vi "Shift_008.vi"() -> ()   [LabVIEW 2019]
uses:
  <vilib>/Utility/file.llb/Write Delimited Spreadsheet (DBL).vi
panel:
  out "path":path
  out "Force Chart":cluster{dbl[unit], dbl[unit]}(graph)
  out "Energies":dbl[unit][][](array[numeric])
  out "Energies":dbl[unit][][](graph)
  in  "time threshold 2":dbl[unit]=5.0
  in  "Control Force 2":dbl[unit]=1000.0
  in  "time threshold 1":dbl[unit]=2.0
  in  "Control Force 1":dbl[unit]=1000.0
  in  "D":dbl[unit]=25.0
  out "Ep(tk)":dbl[unit][](array[numeric])
  out "Et(tk)":dbl[unit][](array[numeric])
  out "Ek(tk)":dbl[unit][](array[numeric])
  out "Et":cluster{dbl[unit][], dbl[unit][]}(graph)
  out "Ep":cluster{dbl[unit][], dbl[unit][]}(graph)
  out "Ek":cluster{dbl[unit][], dbl[unit][]}(graph)
  out "Et":dbl[unit][](graph)
  out "Ep":dbl[unit][](graph)
  out "Ek":dbl[unit][](graph)
  out "a":cluster{dbl[unit][], dbl[unit][]}(graph)
  out "v":cluster{dbl[unit][], dbl[unit][]}(graph)
  out "x":cluster{dbl[unit][], dbl[unit][]}(graph)
  out "time (tk)":dbl[unit][](array[numeric])
  out "a":dbl[unit][](graph)
  out "v":dbl[unit][](graph)
  out "x":dbl[unit][](graph)
  out "x(tk)":dbl[unit][](array[numeric])
  out "v(tk)":dbl[unit][](array[numeric])
  out "a(tk)":dbl[unit][](array[numeric])
  in  "M":dbl[unit]=100.0
  in  "k":dbl[unit]=1000.0
  in  "v0":dbl[unit]
  in  "x0":dbl[unit]=2.0
  in  "Dt":dbl[unit]=1e-05
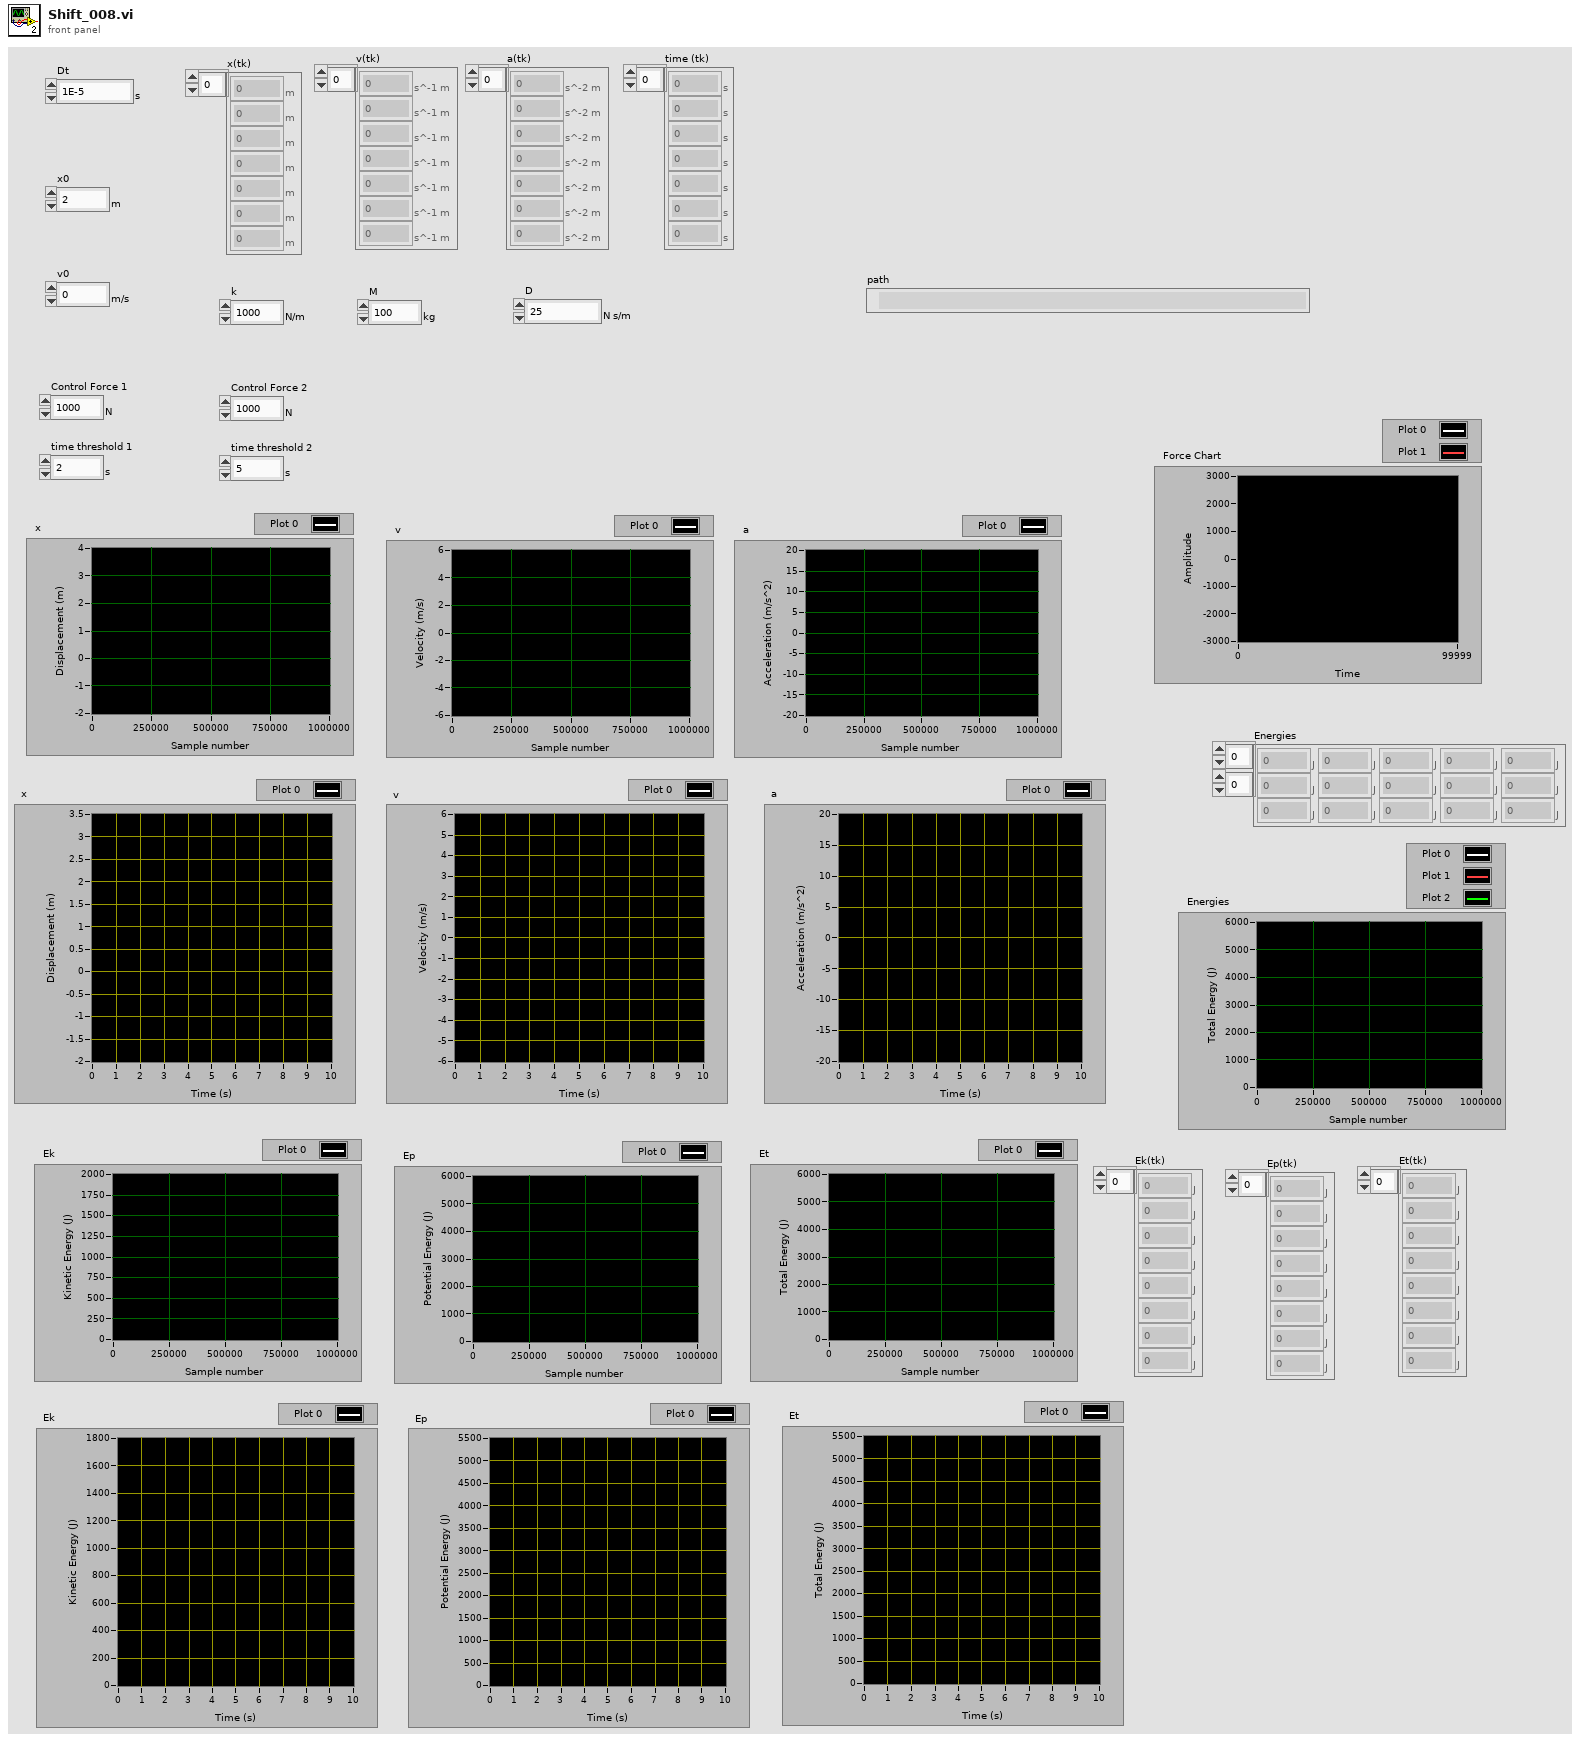
[diagram p1: front panel]
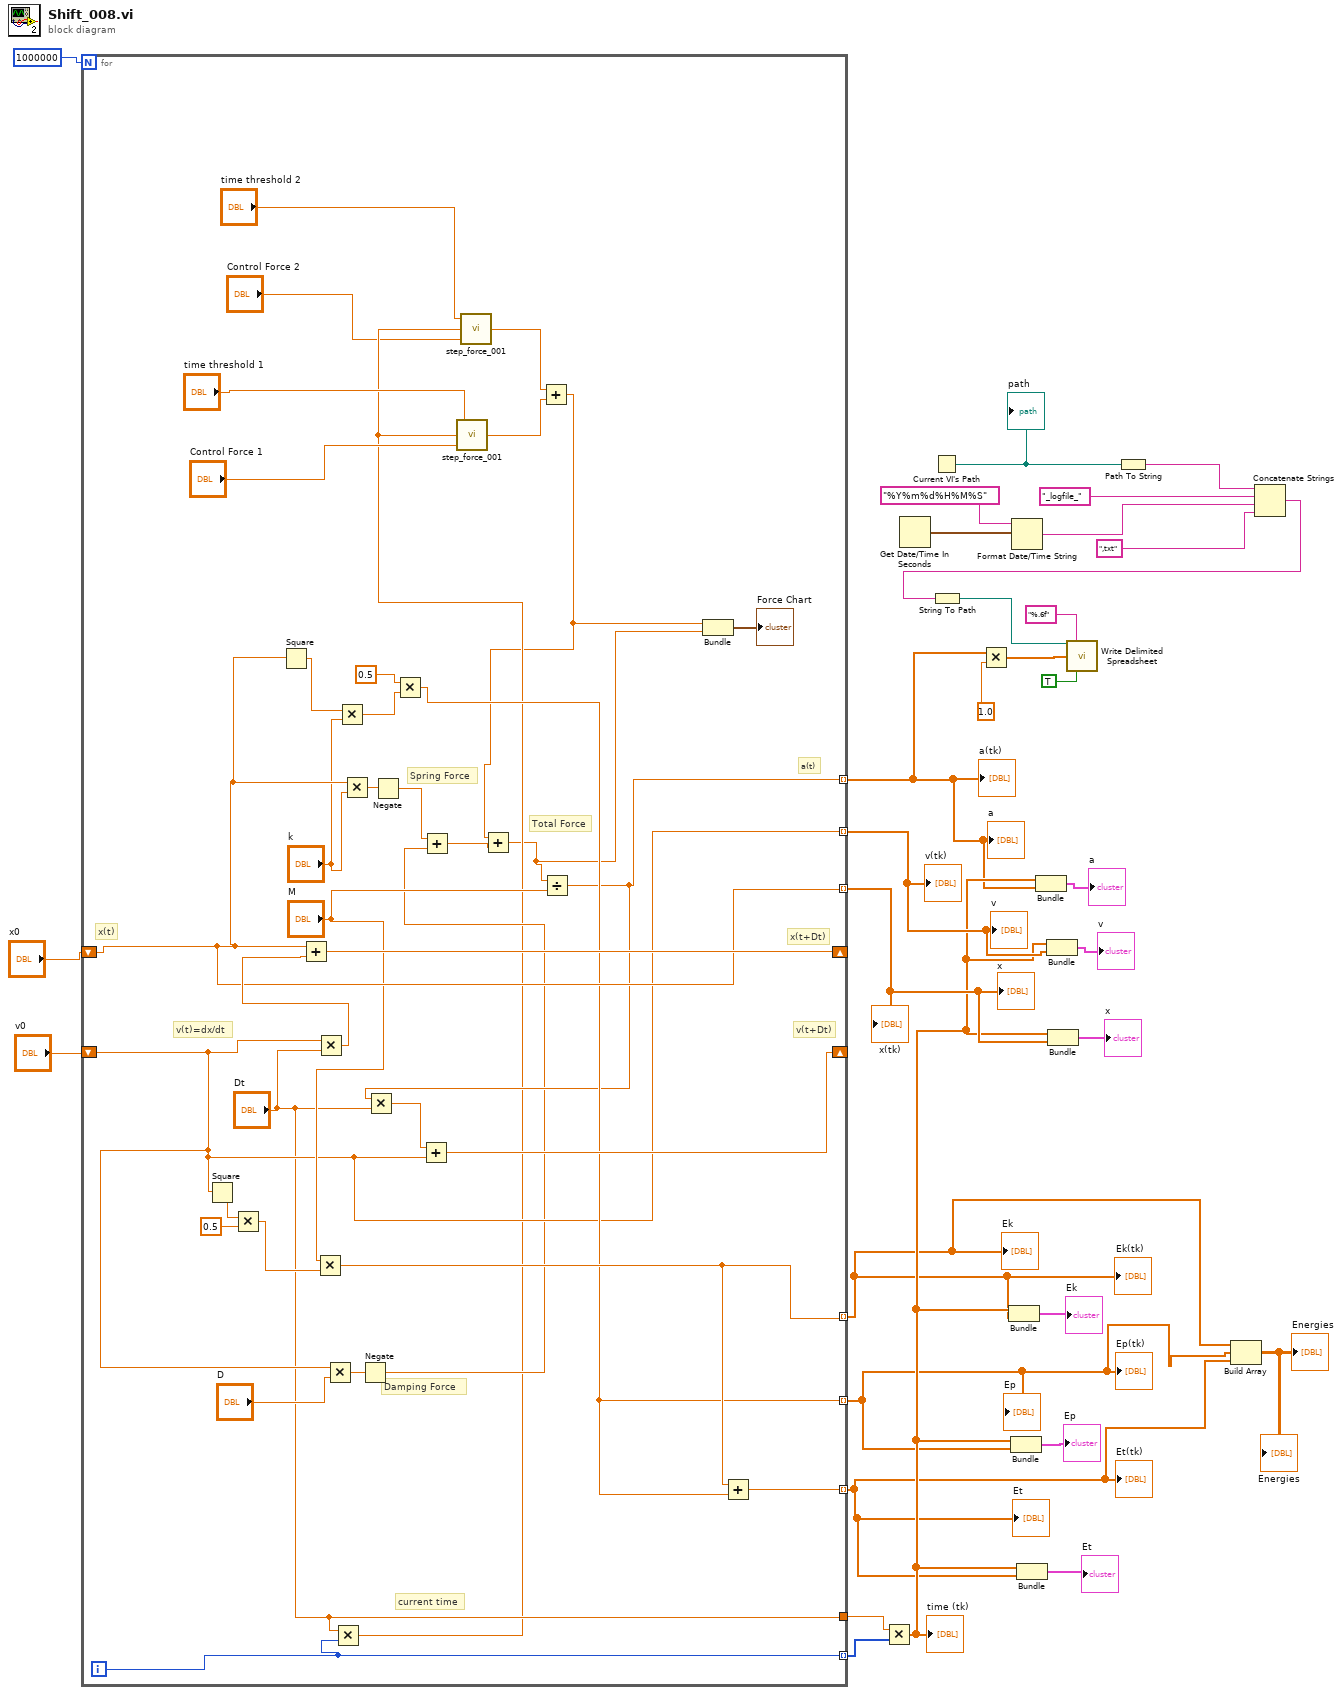
[diagram p0: block diagram]
diagram:
  n1 = for {
    N: 1000000 -> [_]
    shift-right: [w67] -> _
    shift-left: "x0" -> [w61]
    shift-right: [w64] -> _
    shift-left: "v0" -> [w51]
    tunnel: [w47] -> w14 mode=indexing
    tunnel: [w51] -> w24 mode=indexing
    tunnel: [w61] -> w23 mode=indexing
    tunnel: [w43] -> w28 mode=indexing
    tunnel: ["Dt"] -> w29
    tunnel: [w56] -> w18 mode=indexing
    tunnel: [w53] -> w17 mode=indexing
    tunnel: [w55] -> w16 mode=indexing
    i -> [w43]
    # "Total Force"
    # "current time"
    # "Spring Force"
    # "Damping Force"
    # "a(t)"
    # "v(t+Dt)"
    # "x(t+Dt)"
    # "v(t)=dx/dt"
    # "x(t)"
    n2 = Square(x=w51) -> (x^2=w62:dbl[unit])
    n3 = Multiply(x=w62, y=0.5) -> (x*y=w57:dbl[unit])
    n4 = Square(x=w61) -> (x^2=w60:dbl[unit])
    n5 = Multiply(x="M", y=w57) -> (x*y=w56:dbl[unit])
    n6 = Multiply(x=w51, y="Dt") -> (x*y=w68:dbl[unit])
    n7 = Add(x=w61, y=w68) -> (x+y=w67:dbl[unit])
    n8 = Multiply(x=w51, y="D") -> (x*y=w50:dbl[unit])
    n9 = Multiply(x="Dt", y=w43) -> (x*y=w40:dbl[unit])
    n10 = Multiply(x=w60, y="k") -> (x*y=w59:dbl[unit])
    n11 = Multiply(x=w61, y="k") -> (x*y=w66:dbl[unit])
    n12 = Negate(x=w50) -> (-x=w46:dbl[unit])
    n13 = Negate(x=w66) -> (-x=w48:dbl[unit])
    n14 = Multiply(x=0.5, y=w59) -> (x*y=w53:dbl[unit])
    n15 = Add(x=w48, y=w46) -> (x+y=w45:dbl[unit])
    n16 = call "step_force_001.vi"("Control Force in"="Control Force 1", "Current time"=w40, "time threshold"="time threshold 1") -> ("Control Force out"=w37:dbl[unit])
    n17 = call "step_force_001.vi"("Control Force in"="Control Force 2", "Current time"=w40, "time threshold"="time threshold 2") -> ("Control Force out"=w36:dbl[unit])
    n18 = Add(x=w36, y=w37) -> (x+y=w35:dbl[unit])
    n19 = Add(x=w35, y=w45) -> (x+y=w34:dbl[unit])
    n20 = Divide(x=w34, y="M") -> (x/y=w47:dbl[unit])
    n21 = Multiply(x=w47, y="Dt") -> (x*y=w65:dbl[unit])
    n22 = Add(x=w65, y=w51) -> (x+y=w64:dbl[unit])
    n23 = Bundle(w35, w34) -> (→"Force Chart":cluster{dbl[unit], dbl[unit]})  [unwired: 1 in]
    n24 = Add(x=w56, y=w53) -> (x+y=w55:dbl[unit])
  }
  "a(tk)" <- w14
  "v(tk)" <- w24
  "x(tk)" <- w23
  "v" <- w24
  "a" <- w14
  "x" <- w23
  "Et" <- w16
  "Ek" <- w18
  "Ep" <- w17
  "Ek(tk)" <- w18
  "Et(tk)" <- w16
  "Ep(tk)" <- w17
  n25 = Multiply(x=w29, y=w28) -> (x*y=w19:dbl[unit][])
  "time (tk)" <- w19
  n26 = Get Date/Time In Seconds() -> (seconds since 1Jan1904=w8:timestamp)
  n27 = Current VI's Path() -> (path=w2:path)
  "path" <- w2
  n28 = Multiply(x=w14, y=dbl[unit] 1.0 ("Numeric")) -> (x*y=w12:dbl[])
  n29 = Bundle(w19, w18) -> (→"Ek":cluster{dbl[unit][], dbl[unit][]})  [unwired: 1 in]
  n30 = Bundle(w19, w17) -> (→"Ep":cluster{dbl[unit][], dbl[unit][]})  [unwired: 1 in]
  n31 = Format Date/Time String(time format string (%c)="%Y%m%d%H%M%S", seconds (now)=w8) -> (date/time string=w5:string)  [unwired: 1 in]
  n32 = Bundle(w19, w16) -> (→"Et":cluster{dbl[unit][], dbl[unit][]})  [unwired: 1 in]
  n33 = Bundle(w19, w14) -> (→"a":cluster{dbl[unit][], dbl[unit][]})  [unwired: 1 in]
  n34 = Bundle(w19, w24) -> (→"v":cluster{dbl[unit][], dbl[unit][]})  [unwired: 1 in]
  n35 = Bundle(w19, w23) -> (→"x":cluster{dbl[unit][], dbl[unit][]})  [unwired: 1 in]
  n36 = Path To String(path=w2) -> (string=w1:string)
  n37 = Build Array(w18, w17, w16) -> (→"Energies" →"Energies":dbl[unit][][])
  n38 = Concatenate Strings(w1, "_logfile_" ("string"), w5, ",txt" ("string")) -> (w3:string)
  n39 = String To Path(string=w3) -> (path=w9:path)
  n40 = call-poly <vilib>:"Write Delimited Spreadsheet.vi"("file path (dialog if empty)"=w9, "format (%.3f)"="%.6f", "1D data"=w12, "transpose? (no:F)"=TRUE) -> ()  [unwired: 10 in, 2 out]
